vi "both servo with limitation.vi"   [LabVIEW 2010, in "Tank Robot.lvrbt"]
uses:
  Tank Robot.lvrbt
  <vilib>/NXT/Subs/LVHSConnector.ctl
  <vilib>/NXT/NXTIO Xnodes/AddressXNode/NXTIOAddress.xnode
  <vilib>/NXT/Subs/MotorXNode.Servo Type.ctl
  <vilib>/NXT/Subs/MotorXNode.1Servo.ctl
  <vilib>/NXT/NXTIO Xnodes/NXTIOXNode/NXTIO.xnode
  <vilib>/NXT/NXTIO Xnodes/NXTIONodeSubVIs/TETRIX IO Move Servos.vi
types:
  T1 = typedef "MotorXNode.Servo Type.ctl" = enum16{"Servo"}
  T2 = typedef "FTC ControllerState.ctl" = cluster{"Left X":i8, "Left Y":i8, "Right X":i8, "Right Y":i8, "Button Encoding 9-12":u8, "Button Encoding 1-8":u8, "POV":T3}
  T3 = typedef "FTC POVState.ctl" = i8
  T4 = typedef "FTC ButtonState.ctl" = cluster{"Button 1":bool, "Button 2":bool, "Button 3":bool, "Button 4":bool, "Button 5":bool, "Button 6":bool, "Button 7":bool, "Button 8":bool, "Button 9":bool, "Button 10":bool, "Button 11":bool, "Button 12":bool, "POV":T3}
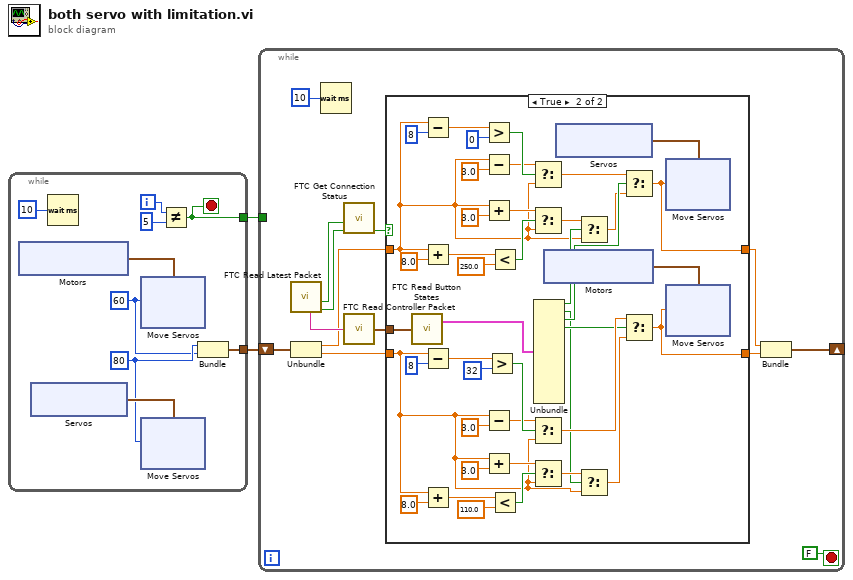
[diagram p0: block diagram]
diagram:
  n1 = while {
    tunnel: [w8] -> w2
    tunnel: [w3] -> w1
    i -> [w11]
    stop <- w8 stop-if-true
    w4 = u8 60 ("Position 1")
    w5 = u8 80 ("Position 1")
    n2 = xnode "Motors"() -> ("Servo"=w6:cluster{"Servo":T1, "Address":i16})
    n3 = xnode "Servos"() -> ("Servo"=w7:cluster{"Servo":T1, "Address":i16})
    n4 = Wait (ms)(milliseconds to wait=u32 10) -> ()  [unwired: 1 out]
    n5 = xnode "Move Servos"("Position 1"=w4, "Servos"=w6) -> ()  [unwired: 1 in, 1 out]
    n6 = xnode "Move Servos"("Position 1"=w5, "Servos"=w7) -> ()  [unwired: 1 in, 1 out]
    n7 = Not Equal?(x=w11, y=5) -> (x != y?=w8:bool)
    n8 = Bundle("Position 1"=w5, "Position 1"=w4) -> (w3:cluster{"Position 1":u8, "Position 1":u8})  [unwired: 1 in]
  }
  n9 = while {
    tunnel: w2 -> [_]
    shift-right: [w30] -> _
    shift-left: w1 -> [w35]
    stop <- FALSE stop-if-true
    n10 = call <vilib>:"FTC Read Latest Packet.vi"() -> ("Packet Received?"=w39:bool, "Stopped?"=w40:bool, "Controller 1"=w37:string)  [unwired: 6 in, 3 out]
    n11 = Unbundle(w35) -> ("Position 1"=w34:dbl, "Position 1"=w33:dbl)
    n12 = Wait (ms)(milliseconds to wait=u32 10) -> ()  [unwired: 1 out]
    n13 = call <vilib>:"FTC Get Connection Status.vi"("Packet Received?"=w39, "Stopped?"=w40) -> ("Online?"=w38:bool)  [unwired: 6 in, 2 out]
    n14 = call <vilib>:"FTC Read Controller Packet.vi"("Packet"=w37) -> ("Controller State"=w36:T2)  [unwired: 4 in]
    n15 = case shown="True" w38 {
      tunnel: w36 -> [_ w86]
      tunnel: w34 -> [w44 w67]
      tunnel: w33 -> [w43 w46]
      tunnel: [w44 w64] -> w32
      tunnel: [w43 w45] -> w31
      frame False {
      }
      frame True {
        n16 = call <vilib>:"FTC Read Button States.vi"("Controller State"=w86) -> ("Button States"=w85:T4)  [unwired: 2 in, 1 out]
        n17 = Subtract(x=w67, y=u8 8) -> (x-y=w82:dbl)
        n18 = Add(x=w67, y=8.0) -> (x+y=w73:dbl)
        n19 = Subtract(x=w46, y=u8 8) -> (x-y=w62:dbl)
        n20 = Add(x=w46, y=8.0) -> (x+y=w55:dbl)
        n21 = Greater?(x=w82, y=u8 0) -> (0:w80:bool)
        n22 = Subtract(x=w67, y=3.0) -> (x-y=w79:dbl)
        n23 = Add(x=w67, y=3.0) -> (x+y=w70:dbl)
        n24 = Subtract(x=w46, y=3.0) -> (x-y=w59:dbl)
        n25 = Add(x=w46, y=3.0) -> (x+y=w52:dbl)
        n26 = Greater?(x=w62, y=u8 32) -> (0:w60:bool)
        n27 = Less?(x=w73, y=250.0) -> (x < y?=w71:bool)
        n28 = Less?(x=w55, y=110.0) -> (x < y?=w53:bool)
        n29 = Select(t=w79, s=w80, f=w67) -> (s? t:f=w77:dbl)
        n30 = Select(t=w70, s=w71, f=w67) -> (s? t:f=w68:dbl)
        n31 = Select(t=w59, s=w60, f=w46) -> (s? t:f=w57:dbl)
        n32 = Select(t=w52, s=w53, f=w46) -> (s? t:f=w50:dbl)
        n33 = Unbundle(w85) -> ("Button 1"=w75:bool, "Button 2"=w47:bool, "Button 3"=w76:bool, "Button 4"=w48:bool)  [unwired: 9 out]
        n34 = xnode "Motors"() -> ("Servo"=w65:cluster{"Servo":T1, "Address":i16})
        n35 = xnode "Servos"() -> ("Servo"=w84:cluster{"Servo":T1, "Address":i16})
        n36 = Select(t=w68, s=w75, f=w67) -> (s? t:f=w66:dbl)
        n37 = Select(t=w50, s=w47, f=w46) -> (s? t:f=w49:dbl)
        n38 = Select(t=w77, s=w76, f=w66) -> (s? t:f=w64:dbl)
        n39 = Select(t=w57, s=w48, f=w49) -> (s? t:f=w45:dbl)
        n40 = xnode "Move Servos"("Position 1"=w64, "Servos"=w84) -> ()  [unwired: 1 in, 1 out]
        n41 = xnode "Move Servos"("Position 1"=w45, "Servos"=w65) -> ()  [unwired: 1 in, 1 out]
      }
    }
    n42 = Bundle("Position 1"=w32, "Position 1"=w31) -> (w30:cluster{"Position 1":dbl, "Position 1":dbl})  [unwired: 1 in]
  }
